vi "Vision Processing.vi"(4 "error in (no error)":errorcluster, 6 "CameraDevRef":T1) -> ()   [LabVIEW 2011]
uses:
  <vilib>/Rock Robotics/WPI/Camera/WPI_CameraDevRef.ctl
  Robot Global Data.vi
  <vilib>/vision/NI_Vision_Development_Module.lvlib
panel:
  in  "Y AbsolVal Difference":dbl=0.25
  in  "Default Shooter Speed Dump":dbl=0.42
  in  "Default Shooter Speed Shoot":dbl=0.705
  in  "Scale":dbl=0.85
  in  "Minimum Power":dbl=0.22
  out "Aspect Ratio":dbl[](array[numeric])
  out "Offset":dbl
  out "Raw Turret":dbl
  out "Target X Coord":dbl
  out "Target Distance":dbl
  out "Distance Array":dbl[](array[numeric])
  in  "Dead Band":dbl=0.09
  out "Number of Rectangles Visible":dbl
  out "Y Position Array":dbl[](array[numeric])
  out "X Position Array":dbl[](array[numeric])
  in  "View":bool
  out "Target Info":T2(array[cluster])
  in  "Area Size Limit":i32=444
  in  "Particle Count Limit":i32=8
  in  "Score Limits":T3={"Rect Coverage"=76.0, "Aspect Ratio"=40.0, "X Edge Strength"=40.0, "Y Edge Strength"=60.0}
  in  "Processing":enum32{"Color", "Intensity", "Intensity Open"}(tab)=enum."Intensity"
  in  "Luminance":i32=255
  in  "Saturation":i32=255
  in  "Hue":i32(knob)=65 scale=0.0..255.0
  in  "Margins":cluster{"Hue":i32, "Sat":i32, "Lum":i32}={"Hue"=20, "Sat"=27, "Lum"=30} {"Sat" scale=0.0..40.0; "Lum" scale=0.0..40.0; "Hue" scale=0.0..40.0}
  in  "Range":cluster{"Lower value":sgl, "Upper value":sgl}={"Lower value"=151.52174, "Upper value"=255.0} {"Lower value" scale=0.0..255.0; "Upper value" scale=0.0..255.0}
  in  "Range":cluster{"Lower value":sgl, "Upper value":sgl}={"Lower value"=123.804344, "Upper value"=255.0} {"Lower value" scale=0.0..255.0; "Upper value" scale=0.0..255.0}
  in  "View":bool
  out "Processed Image":T4(plugin-control)
  out "Original Image":T4(plugin-control)
  # "Instructions:\nProcessing the reflective tape that is illuminated by a ring light can be based\non color or light intensity.\nParticles within the image are scored by rectangle coverage, aspect ratio, and\nfor being hollow with a bold edge. A particle is considered a target if all scores\nare above the score limits. Particles can be annotated -- surrounded by\na rectangle and scores drawn to the left .\nTo control the number of particles being scored, use the count limit and the size\nlimit."
  # "(in)"
  # "To debug, Enable using the View button.\nFor color processing, you can click in the image to select the color for processing."
  # "Enable by clicking the View button.\nGreen scores are above the limit, orange are below. Inner/outer rect\nindicates all passed."
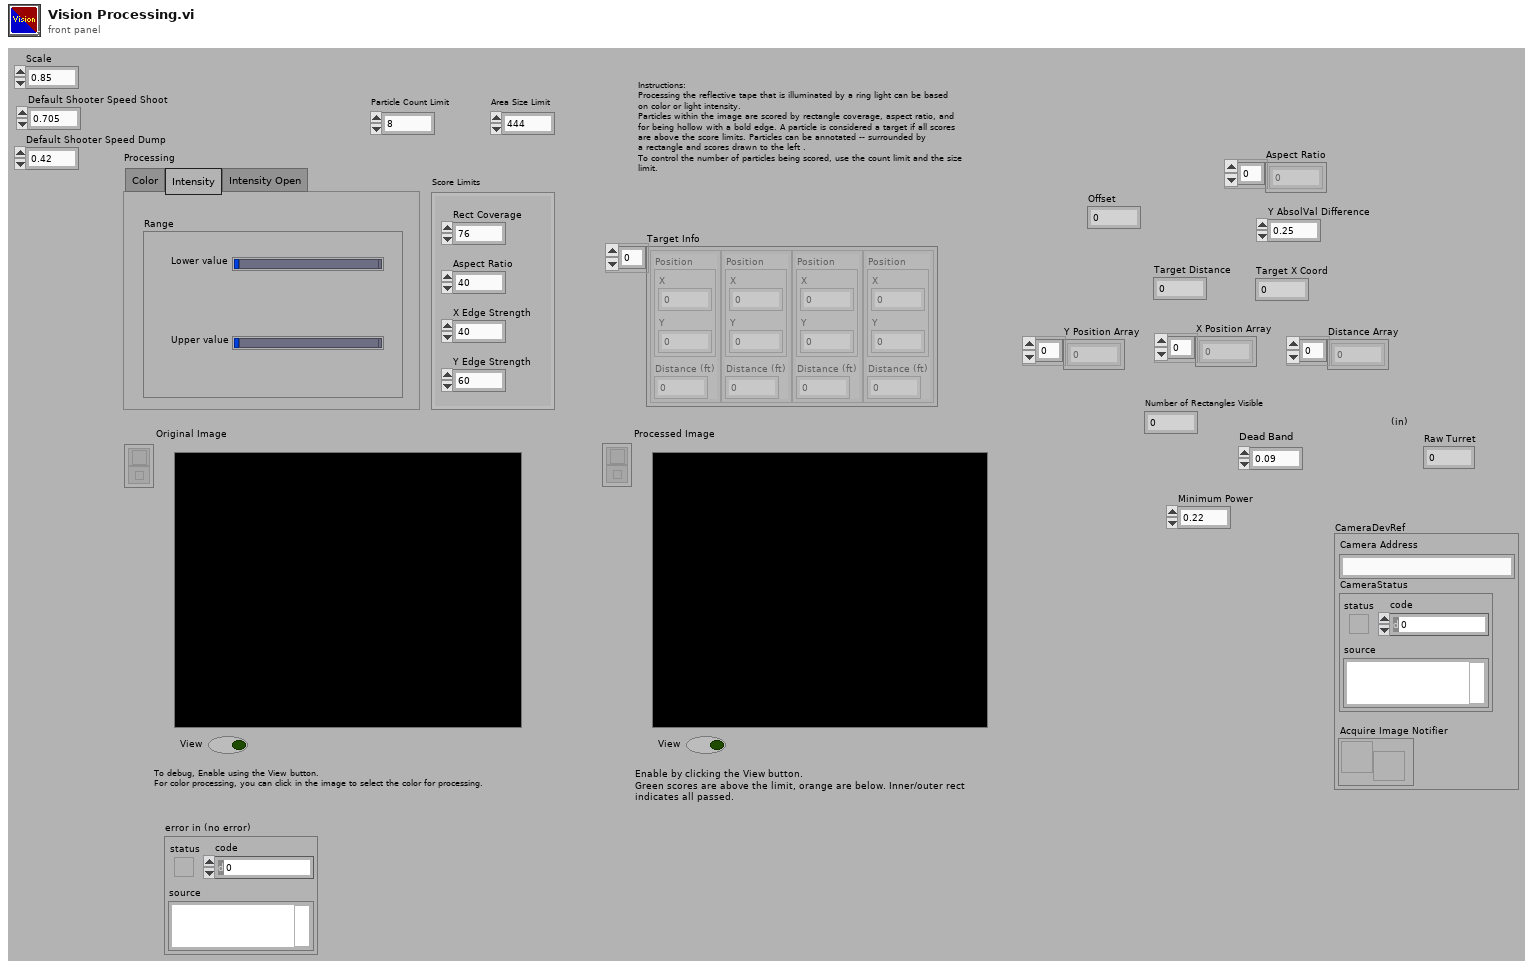
[diagram p1: front panel]
types:
  T1 = typedef "WPI_CameraDevRef.ctl" = cluster{"Camera Address":string, "CameraStatus":errorcluster, "Acquire Image Notifier":refnum<notifier>}
  T2 = cluster{"Position":cluster{"X":dbl, "Y":dbl}, "Distance (ft)":dbl}[]
  T3 = cluster{"Rect Coverage":dbl, "Aspect Ratio":dbl, "X Edge Strength":dbl, "Y Edge Strength":dbl}
  T4 = typedef "IMAQ Image.ctl" = refnum<image>
  T5 = typedef "Image Type" = u32
  T6 = enum32{"AutoM", "Close", "Dilate", "Erode", "Gradient", "Gradient out", "Gradient in", "Hit miss", "Open", "PClose", "POpen", "Thick", "Thin"}
  T7 = typedef "WPI_CameraImageSize.ctl" = enum16{"640x480", "320x240", "160x120"}
  T8 = cluster{"fps":i32, "compression":i32, "Image Size":T7}
  T9 = cluster{cluster{"Left":dbl, "Top":dbl, "Right":dbl, "Bottom":dbl}, dbl[]}[]
  T10 = cluster{"Left":dbl, "Top":dbl, "Right":dbl, "Bottom":dbl}
  T11 = cluster{"Target Center (-1 to 1)":cluster{"X":dbl, "Y":dbl}, "Distance (ft)":dbl}
  T12 = cluster{"Target Center (-1 to 1)":cluster{"X":dbl, "Y":dbl}, "Distance (ft)":dbl}[]
  T13 = typedef "WPI_JoystickDevRef.ctl" = cluster{"Device":T14}
  T14 = typedef "WPI_JoystickDeviceEnum.ctl" = enum16{"USB 1", "USB 2", "USB 3", "USB 4", "Kinect 1", "Kinect 2"}
  T15 = typedef "WPI_JoystickButtonState.ctl" = cluster{"Button 1":bool, "Button 2":bool, "Button 3":bool, "Button 4":bool, "Button 5":bool, "Button 6":bool, "Button 7":bool, "Button 8":bool, "Button 9":bool, "Button 10":bool, "Button 11":bool, "Button 12":bool}
  T16 = cluster{"axis 1 (x)":dbl, "axis 2 (y)":dbl, "axis 3 (throttle)":dbl, "axis 4":dbl, "axis 5":dbl, "axis 6":dbl}
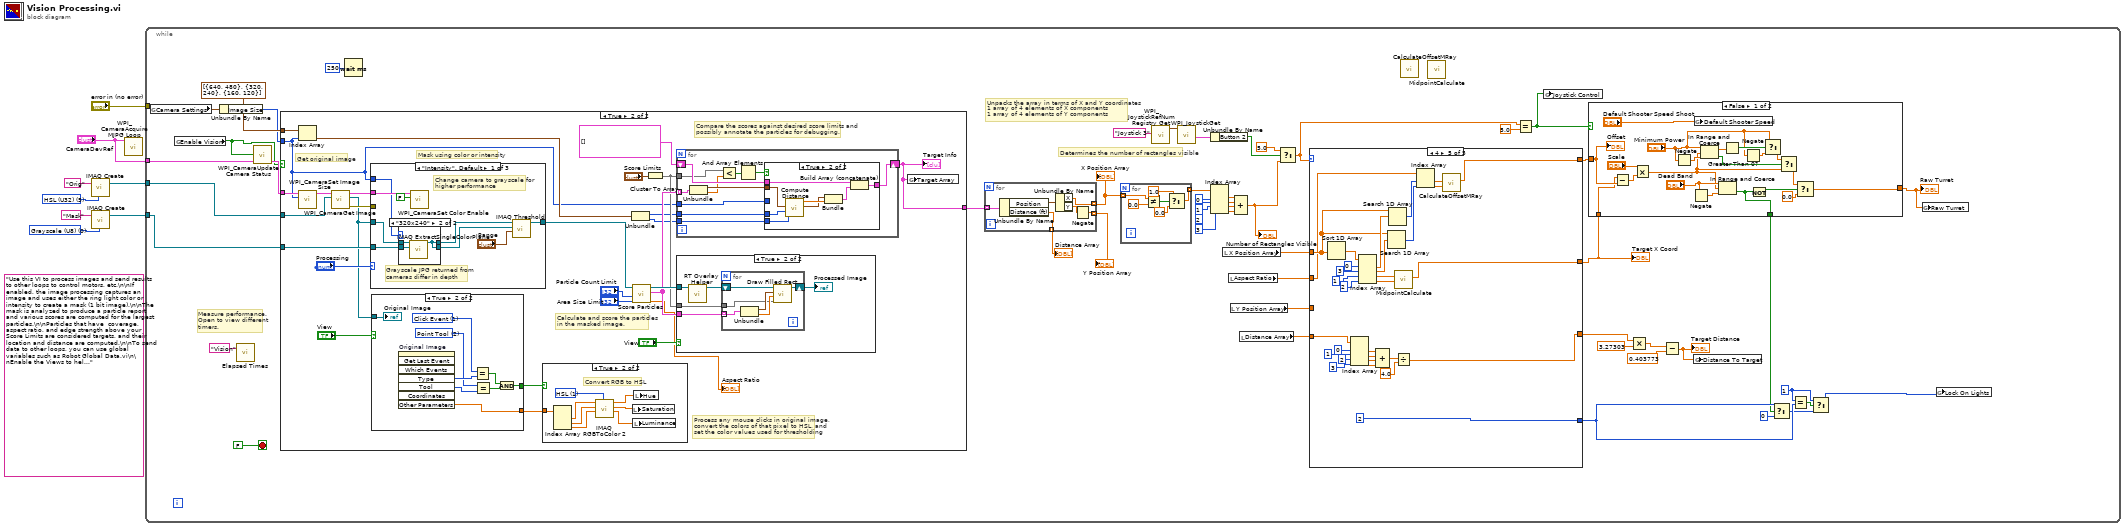
[diagram p0: block diagram]
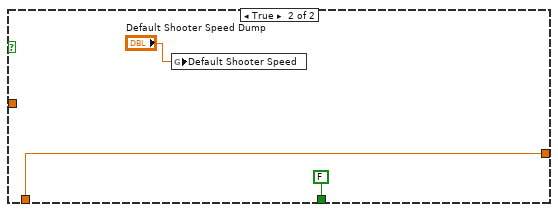
[diagram p2: hidden frame]
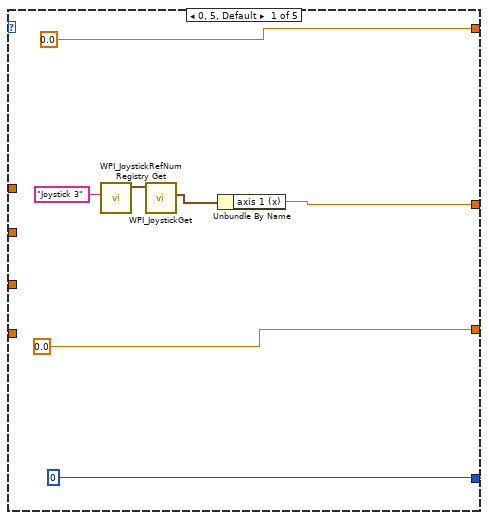
[diagram p3: hidden frame]
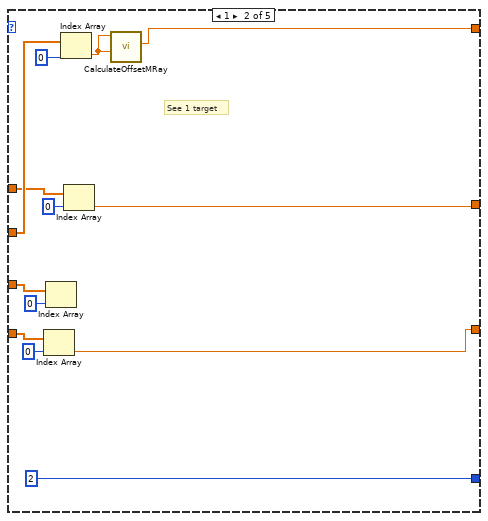
[diagram p4: hidden frame]
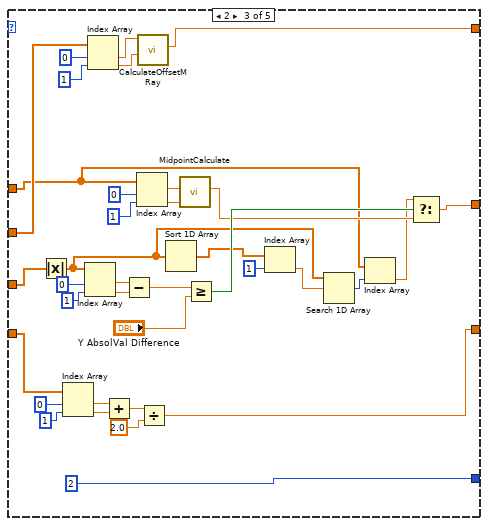
[diagram p5: hidden frame]
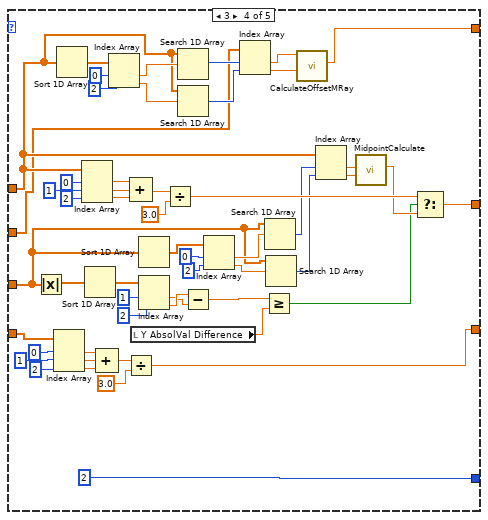
[diagram p6: hidden frame]
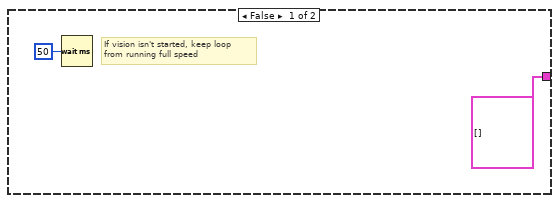
[diagram p7: hidden frame]
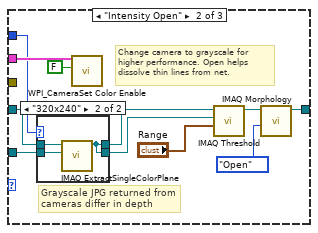
[diagram p10: hidden frame]
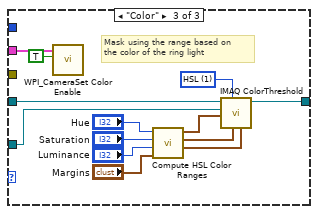
[diagram p12: hidden frame]
diagram:
  w3 = T5 0 items=["Grayscale (U8)", "Grayscale (I16)", "Grayscale (SGL)", "Complex (CSG)", "RGB (U32)", "HSL (U32)", "RGB (U64)", "Grayscale (U16)"] ("Image Type")
  (unwired) "Use this VI to process images and send results to other loops to control motors, etc.\n\nIf enabled, the image processing captures an image and uses either the ring light color or intensity to create a mask (1 bit image).\n\nThe mask is analyzed to produce a particle report and various scores are computed for the largest particles.\n\nParticles that have  coverage, aspect ratio, and edge strength above your Score Limits are considered targets, and their location and distance are computed.\n\nTo send data to other loops, you can use global variables such as Robot Global Data.vi\n\nEnable the Views to help debug color settings. Disable the View to speed up processing."
  w7 = T5 5 items=["Grayscale (U8)", "Grayscale (I16)", "Grayscale (SGL)", "Complex (CSG)", "RGB (U32)", "HSL (U32)", "RGB (U64)", "Grayscale (U16)"] ("Image Type")
  n1 = call "IMAQ Create"("Image Name"="Orig", "Image Type"=w7) -> ("New Image"=w6:T4)  [unwired: 2 in, 2 out]
  n2 = call "IMAQ Create"("Image Name"="Mask", "Image Type"=w3) -> ("New Image"=w1:T4)  [unwired: 2 in, 2 out]
  n3 = call <vilib>:"WPI_CameraAcquire MJPG Loop.vi"("CameraDevRef"="CameraDevRef") -> ()  [unwired: 11 in]
  n4 = while {
    tunnel: w6 -> [w59]
    tunnel: "CameraDevRef" -> [w58]
    tunnel: "error in (no error)" -> [_]
    tunnel: w1 -> [w54]
    stop <- FALSE stop-if-true
    w24 = 1 ("y")
    # "Determines the number of rectangles visible"
    # "Unpacks the array in terms of X and Y coordinates\n1 array of 4 elements of X components\n1 array of 4 elements of Y components"
    # "Measure performance.\nOpen to view different\ntimers."
    n5 = global read "Robot Global Data.vi" "Camera Settings"() -> (w52:T8)
    n6 = global read "Robot Global Data.vi" "Enable Vision"() -> (w56:bool)
    n7 = Unbundle By Name(w52) -> ("Image Size"=w51:T7)
    n8 = call "Elapsed Times.vi"("Call Name"="Vision") -> ()  [unwired: 2 in, 1 out]
    n9 = call <vilib>:"WPI_CameraUpdate Camera Status.vi"("CameraDevRef In"=w58, "Enable Vision"=w56) -> ("CameraDevRef Out"=w57:T1)  [unwired: 3 in]
    n10 = case shown="True" w56 {
      tunnel: w59 -> [_ w254]
      tunnel: w57 -> [_ w250]
      tunnel: w54 -> [_ w241]
      tunnel: cluster{i32, i32}[] [{640, 480}, {320, 240}, {160, 120}] -> [_ w245]
      tunnel: w51 -> [_ w238]
      tunnel: [T2 [] w239] -> w50
      frame False {
        # "If vision isn't started, keep loop\nfrom running full speed"
        n11 = Wait (ms)(milliseconds to wait=u32 50) -> ()  [unwired: 1 out]
      }
      frame True {
        # "Compare the scores against desired score limits and\npossibly annotate the particles for debugging."
        # "Process any mouse clicks in original image,\nconvert the colors of that pixel to HSL, and\nset the color values used for thresholding"
        # "Calculate and score the particles\nin the masked image."
        # "Mask using color or intensity"
        # "Get original image"
        n12 = call <vilib>:"WPI_CameraSet Image Size.vi"("Image Size"=w238, "CameraDevRef"=w250) -> ("CameraDevRef Out"=w251:T1)  [unwired: 8 in, 1 out]
        n13 = Index Array(array=w245, index=w238) -> (element=w242:cluster{i32, i32})
        n14 = call <vilib>:"WPI_CameraGet Image.vi"("Image"=w254, "CameraDevRef"=w251) -> ("error out"=w252:errorcluster, "Image Out"=w240:T4, "CameraDevRef Out"=w253:T1)  [unwired: 7 in]
        n15 = case shown="\"Intensity\", Default" "Processing" {
          tunnel: w240 -> [w276 w288 w314]
          tunnel: [w279 w293 w313] -> w248
          tunnel: w253 -> [w277 w291 w304]
          tunnel: w252 -> [_ _ _]
          tunnel: w241 -> [w275 w289 w302]
          tunnel: w238 -> [w274 w290 _]
          frame "Intensity", Default {
            # "Grayscale JPG returned from\ncameras differ in depth"
            # "Change camera to grayscale for\nhigher performance"
            n16 = case shown="\"320x240\"" w274 {
              tunnel: w276 -> [w282 w285]
              tunnel: w275 -> [w281 w284]
              tunnel: [w282 w283] -> w273
              tunnel: [w281 w283] -> w272
              frame "640x480", Default {
              }
              frame "320x240" {
                n17 = call "IMAQ ExtractSingleColorPlane"("Image Dst"=w284, "Image Src"=w285) -> ("Image Dst Out"=w283:T4)  [unwired: 8 in, 1 out]
              }
            }
            n18 = call <vilib>:"WPI_CameraSet Color Enable.vi"("Color Enabled"=FALSE, "CameraDevRef"=w277) -> ()  [unwired: 8 in, 2 out]
            n19 = call "IMAQ Threshold"("Range"="Range", "Image Dst"=w272, "Image Src"=w273) -> ("Image Dst Out"=w279:T4)  [unwired: 3 in, 5 out]
          }
          frame "Intensity Open" {
            # "Grayscale JPG returned from\ncameras differ in depth"
            # "Change camera to grayscale for\nhigher performance. Open helps\ndissolve thin lines from net."
            n20 = case shown="\"320x240\"" w290 {
              tunnel: w288 -> [w298 w301]
              tunnel: w289 -> [w297 w300]
              tunnel: [w298 w299] -> w287
              tunnel: [w297 w299] -> w286
              frame "640x480", Default {
              }
              frame "320x240" {
                n21 = call "IMAQ ExtractSingleColorPlane"("Image Dst"=w300, "Image Src"=w301) -> ("Image Dst Out"=w299:T4)  [unwired: 8 in, 1 out]
              }
            }
            n22 = call <vilib>:"WPI_CameraSet Color Enable.vi"("Color Enabled"=FALSE, "CameraDevRef"=w291) -> ()  [unwired: 8 in, 2 out]
            n23 = call "IMAQ Threshold"("Range"="Range", "Image Dst"=w286, "Image Src"=w287) -> ("Image Dst Out"=w294:T4)  [unwired: 3 in, 5 out]
            n24 = call "IMAQ Morphology"("Operation"=T6."Open", "Image Src"=w294) -> ("Image Dst Out"=w293:T4)  [unwired: 8 in, 1 out]
          }
          frame "Color" {
            w312 = u16 1 items=["RGB", "HSL", "HSV", "HSI"] ("Color Mode")
            # "Mask using the range based on\nthe color of the ring light"
            n25 = call <vilib>:"WPI_CameraSet Color Enable.vi"("Color Enabled"=TRUE, "CameraDevRef"=w304) -> ()  [unwired: 8 in, 2 out]
            n26 = call "Compute HSL Color Ranges.vi"("Margins"="Margins", "Luminance"="Luminance", "Saturation"="Saturation", "Hue"="Hue") -> ("Lum Range"=w309:cluster{i32, i32}, "Sat Range"=w310:cluster{i32, i32}, "Hue Range"=w311:cluster{i32, i32})  [unwired: 5 in]
            n27 = call "IMAQ ColorThreshold"("Blue or Luma or Val or Inten Range"=w309, "Green or Sat Range"=w310, "Color Mode"=w312, "Red or Hue Range"=w311, "Image Dst"=w302, "Image Src"=w314) -> ("Image Dst Out"=w313:T4)  [unwired: 4 in, 1 out]
          }
        }
        n28 = case shown="True" "View" {
          tunnel: w240 -> [_ w334]
          tunnel: [_ w329] -> w247
          tunnel: [_ w326] -> w246
          frame False {
          }
          frame True {
            w327 = 2 items=["None", "Selection Tool", "Point Tool", "Line Tool", "Rectangle Tool", "Oval Tool", "Polygon Tool", "ClosedFreehandTool", "Annulus Tool", "Rotated Rectangle Tool", "Zoom Tool", "Pan Tool", "Polyline Tool", "Freehand Tool"] ("Tool")
            w328 = 1 items=["No Event"=0, "Click Event"=1, "Draw Event"=2, "Size Event"=4, "Scroll Event"=5, "Double Click Event"=8] ("Type")
            n29 = invoke on="Original Image" class="ImageControl" method="Get Last Event"() -> ("Type"=w330:i32, "Tool"=w333:i32, "Other Parameters"=w326:sgl[])  [unwired: 8 in, 5 out]
            n30 = Equal?(x=w328, y=w330) -> (x = y?=w331:bool)
            n31 = Equal?(x=w327, y=w333) -> (x = y?=w332:bool)
            n32 = And(x=w331, y=w332) -> (x .and. y?=w329:bool)
            "Original Image" <- w334
          }
        }
        n33 = case shown="True" w247 {
          tunnel: w246 -> [_ w271]
          frame False {
          }
          frame True {
            w270 = u16 1 items=["RGB", "HSL", "HSV", "HSI", "CIE L*a*b*", "CIE XYZ"] ("Color Mode")
            # "Convert RGB to HSL"
            n34 = Index Array(array=w271) -> (element #1=w269:sgl, element #2=w267:sgl, element #3=w265:sgl)  [unwired: 3 in]
            n35 = call "IMAQ RGBToColor 2"("Color Mode"=w270, "Blue value"=w265, "Green value"=w267, "Red value"=w269) -> ("Blue or Luma or Val or Inten or Z or b*value"=w264:dbl, "Green or Sat or Y or a* value"=w266:dbl, "Red or Hue or X or L* value"=w268:dbl)  [unwired: 4 in, 1 out]
            n36 = local write "Saturation"(w266) -> ()
            n37 = local write "Luminance"(w264) -> ()
            n38 = local write "Hue"(w268) -> ()
          }
        }
        n39 = Unbundle(w242) -> (w244:i32, w243:i32)
        n40 = call "Score Particles.vi"("Area Size Limit"="Area Size Limit", "Particle Count Limit"="Particle Count Limit", "Image Refnum in"=w248) -> ("Aspect Ratio"=→"Aspect Ratio":dbl[], "Scored Particle Info"=w259:T9, "Image Refnum out"=w262:T4)  [unwired: 6 in]
        n41 = Cluster To Array(cluster="Score Limits") -> (array=w257:dbl[])
        n42 = for {
          shift-right: [w344] -> w239
          shift-left: T2 [] -> [w345]
          tunnel: w244 -> [w343]
          tunnel: w259 -> [w341] mode=indexing
          tunnel: w257 -> [w336]
          tunnel: w238 -> [w340]
          tunnel: w243 -> [w335]
          n43 = Unbundle(w341) -> (w342:T10, w337:dbl[])
          n44 = Less?(x=w336, y=w337) -> (x < y?=w339:bool[])
          n45 = And Array Elements(Boolean array=w339) -> (logical AND=w338:bool)
          n46 = case shown="True" w338 {
            tunnel: w345 -> [w346 w354]
            tunnel: [w346 w353] -> w344
            tunnel: w342 -> [_ w349]
            tunnel: w343 -> [_ w351]
            tunnel: w340 -> [_ _]
            tunnel: w335 -> [_ w348]
            frame False {
            }
            frame True {
              n47 = call "Compute Distance.vi"("Y Image Resolution"=w348, "X Image Resolution"=w351, "Bounding Box"=w349) -> ("Target Center (-1 to 1)"=w347:cluster{"X":dbl, "Y":dbl}, "Distance (ft)"=w350:dbl)  [unwired: 7 in]
              n48 = Bundle("Target Center (-1 to 1)"=w347, "Distance (ft)"=w350) -> (w352:T11)  [unwired: 1 in]
              n49 = Build Array (concatenate)(w354, w352) -> (w353:T12)
            }
          }
        }
        "Target Info" <- w239
        n50 = case shown="True" "View" {
          tunnel: w262 -> [_ w316]
          tunnel: w259 -> [_ w318]
          tunnel: w257 -> [_ w317]
          frame False {
          }
          frame True {
            n51 = call "RT Overlay Helper.vi"("Refnum in"=w316) -> ("Refnum out"=w319:T4)  [unwired: 10 in]
            n52 = for {
              shift-right: [w324] -> w315
              shift-left: w319 -> [w325]
              tunnel: w318 -> [w321] mode=indexing
              tunnel: w317 -> [w320]
              n53 = Unbundle(w321) -> (w322:T10, w323:dbl[])
              n54 = call "Draw Filled Rect.vi"("Limits"=w320, "Scores"=w323, "Bounding Box"=w322, "image in"=w325) -> ("image out"=w324:T4)  [unwired: 7 in]
            }
            "Processed Image" <- w315
          }
        }
        n55 = global write "Robot Global Data.vi" "Target Array"(w239) -> ()
      }
    }
    n56 = Wait (ms)(milliseconds to wait=u32 250) -> ()  [unwired: 1 out]
    n57 = for {
      tunnel: [w232] -> w30 mode=indexing
      tunnel: [w233] -> w40 mode=indexing
      tunnel: w50 -> [w230] mode=indexing
      tunnel: [w229] -> w42 mode=indexing
      n58 = Unbundle By Name(w230) -> ("Position"=w234:cluster{"X":dbl, "Y":dbl}, "Distance (ft)"=w229:dbl)
      n59 = Unbundle By Name(w234) -> ("X"=w233:dbl, "Y"=w231:dbl)
      n60 = Negate(x=w231) -> (-x=w232:dbl)
    }
    "X Position Array" <- w40
    "Y Position Array" <- w30
    "Distance Array" <- w42
    n61 = for {
      tunnel: w40 -> [w88] mode=indexing
      tunnel: [w84] -> w39 mode=indexing
      n62 = Not Equal?(x=w88, y=0.0) -> (x != y?=w87:bool)
      n63 = Select(t=1.0, s=w87, f=0.0) -> (s? t:f=w84:dbl)
    }
    n64 = call <vilib>:"WPI_JoystickRefNum Registry Get.vi"("refnum name"="Joystick 3") -> ("JoystickDevRef"=w29:T13)  [unwired: 9 in, 1 out]
    n65 = call <vilib>:"WPI_JoystickGet.vi"("JoystickDevRef"=w29) -> ("Buttons"=w27:T15)  [unwired: 4 in, 2 out]
    n66 = Unbundle By Name(w27) -> ("Button 2"=w26:bool)
    n67 = Index Array(array=w39, index #1=0 ("index"), index #2=1 ("index"), index #3=2 ("index"), index #4=3 ("index")) -> (element #1=w37:dbl, element #2=w38:dbl, element #3=w36:dbl, element #4=w35:dbl)
    n68 = local read "X Position Array"() -> (w41:dbl[])
    n69 = local read "Aspect Ratio"() -> (w19:dbl[])
    n70 = local read "Y Position Array"() -> (w43:dbl[])
    n71 = Compound Arithmetic op=ADD(w37, w38, w36, w35) -> (w20:dbl)
    "Number of Rectangles Visible" <- w20
    n72 = local read "Distance Array"() -> (w44:dbl[])
    n73 = Select(t=5.0, s=w26, f=w20) -> (s? t:f=w14:dbl)
    n74 = case shown="4" w14 {
      tunnel: w41 -> [_ w104 w111 w153 w204]
      tunnel: [w92 w103 w135 w187 w227] -> w17
      tunnel: w43 -> [_ w101 w134 w165 _]
      tunnel: w44 -> [_ w99 w123 w196 w224]
      tunnel: [0 2 2 2 2] -> w23
      tunnel: [0.0 ("Offset") w106 w140 w146 w213] -> w18
      tunnel: w19 -> [_ w109 w143 w149 w199]
      tunnel: [0.0 w98 w118 w189 w214] -> w9
      frame 0, 5, Default {
        n75 = call <vilib>:"WPI_JoystickRefNum Registry Get.vi"("refnum name"="Joystick 3") -> ("JoystickDevRef"=w91:T13)  [unwired: 9 in, 1 out]
        n76 = call <vilib>:"WPI_JoystickGet.vi"("JoystickDevRef"=w91) -> ("Axes"=w93:T16)  [unwired: 4 in, 2 out]
        n77 = Unbundle By Name(w93) -> ("axis 1 (x)"=w92:dbl)
      }
      frame 1 {
        # "See 1 target"
        n78 = Index Array(array=w99, index=0) -> (element=w98:dbl)
        n79 = Index Array(array=w101, index=0) -> ()  [unwired: 1 out]
        n80 = Index Array(array=w109, index=0) -> (element=w107:dbl)
        n81 = Index Array(array=w104, index=0) -> (element=w103:dbl)
        n82 = call "CalculateOffsetMRay.vi"("AR2"=w107, "AR1"=w107) -> ("Offset"=w106:dbl)  [unwired: 9 in]
      }
      frame 2 {
        n83 = Absolute Value(x=w134) -> (abs(x)=w114:dbl[])
        n84 = Index Array(array=w123, index #1=0 ("index"), index #2=1 ("index")) -> (element #1=w121:dbl, element #2=w122:dbl)
        n85 = Index Array(array=w114, index #1=0 ("index"), index #2=1 ("index")) -> (element #1=w130:dbl, element #2=w131:dbl)
        n86 = Index Array(array=w143, index #1=0 ("index"), index #2=1 ("index")) -> (element #1=w142:dbl, element #2=w141:dbl)
        n87 = Add(x=w121, y=w122) -> (x+y=w120:dbl)
        n88 = Subtract(x=w130, y=w131) -> (x-y=w129:dbl)
        n89 = Index Array(array=w111, index #1=0 ("index"), index #2=1 ("index")) -> (element #1=w136:dbl, element #2=w137:dbl)
        n90 = call "CalculateOffsetMRay.vi"("AR2"=w141, "AR1"=w142) -> ("Offset"=w140:dbl)  [unwired: 9 in]
        n91 = Divide(x=w120, y=2.0) -> (x/y=w118:dbl)
        n92 = Sort 1D Array(array=w114) -> (sorted array=w116:dbl[])
        n93 = call "MidpointCalculate.vi"("X2"=w137, "X1"=w136) -> ("Midpoint"=w126:dbl)  [unwired: 9 in]
        n94 = Greater Or Equal?(x=w129, y="Y AbsolVal Difference") -> (x >= y?=w127:bool)
        n95 = Index Array(array=w116, index=1) -> (element=w113:dbl)
        n96 = Search 1D Array(1D array=w114, element=w113) -> (index of element=w112:i32)  [unwired: 1 in]
        n97 = Index Array(array=w111, index=w112) -> (element=w110:dbl)
        n98 = Select(t=w110, s=w127, f=w126) -> (s? t:f=w135:dbl)
      }
      frame 3 {
        n99 = Absolute Value(x=w165) -> (abs(x)=w186:dbl[])
        n100 = Index Array(array=w196, index #1=0 ("index"), index #2=1 ("index"), index #3=2 ("index")) -> (element #1=w192:dbl, element #2=w193:dbl, element #3=w194:dbl)
        n101 = Sort 1D Array(array=w153) -> (sorted array=w157:dbl[])
        n102 = Index Array(array=w153, index #1=0 ("index"), index #2=1 ("index"), index #3=2 ("index")) -> (element #1=w174:dbl, element #2=w176:dbl, element #3=w175:dbl)
        n103 = Sort 1D Array(array=w186) -> (sorted array=w170:dbl[])
        n104 = Compound Arithmetic op=ADD(w192, w193, w194) -> (w191:dbl)
        n105 = Index Array(array=w157, index #1=0 ("index"), index #2=2 ("index")) -> (element #1=w154:dbl, element #2=w152:dbl)
        n106 = Divide(x=w191, y=3.0) -> (x/y=w189:dbl)
        n107 = Compound Arithmetic op=ADD(w174, w176, w175) -> (w173:dbl)
        n108 = local read "Y AbsolVal Difference"() -> (w180:dbl)
        n109 = Sort 1D Array(array=w165) -> (sorted array=w169:dbl[])
        n110 = Index Array(array=w170, index #1=1 ("index"), index #2=2 ("index")) -> (element #1=w182:dbl, element #2=w183:dbl)
        n111 = Divide(x=w173, y=3.0) -> (x/y=w171:dbl)
        n112 = Search 1D Array(1D array=w153, element=w154) -> (index of element=w151:i32)  [unwired: 1 in]
        n113 = Search 1D Array(1D array=w153, element=w152) -> (index of element=w150:i32)  [unwired: 1 in]
        n114 = Subtract(x=w183, y=w182) -> (x-y=w181:dbl)
        n115 = Index Array(array=w169, index #1=0 ("index"), index #2=2 ("index")) -> (element #1=w166:dbl, element #2=w164:dbl)
        n116 = Index Array(array=w149, index #1=w151, index #2=w150) -> (element #1=w148:dbl, element #2=w147:dbl)
        n117 = Greater Or Equal?(x=w181, y=w180) -> (x >= y?=w158:bool)
        n118 = Search 1D Array(1D array=w165, element=w166) -> (index of element=w163:i32)  [unwired: 1 in]
        n119 = Search 1D Array(1D array=w165, element=w164) -> (index of element=w162:i32)  [unwired: 1 in]
        n120 = call "CalculateOffsetMRay.vi"("AR2"=w147, "AR1"=w148) -> ("Offset"=w146:dbl)  [unwired: 9 in]
        n121 = Index Array(array=w153, index #1=w163, index #2=w162) -> (element #1=w160:dbl, element #2=w161:dbl)
        n122 = call "MidpointCalculate.vi"("X2"=w161, "X1"=w160) -> ("Midpoint"=w159:dbl)  [unwired: 9 in]
        n123 = Select(t=w171, s=w158, f=w159) -> (s? t:f=w187:dbl)
      }
      frame 4 {
        n124 = Sort 1D Array(array=w204) -> (sorted array=w228:dbl[])
        n125 = Index Array(array=w224, index #1=0 ("index"), index #2=1 ("index"), index #3=2 ("index"), index #4=3 ("index")) -> (element #1=w221:dbl, element #2=w220:dbl, element #3=w219:dbl, element #4=w218:dbl)
        n126 = Index Array(array=w228, index #1=0 ("index"), index #2=3 ("index"), index #3=1 ("index"), index #4=2 ("index")) -> (element #1=w205:dbl, element #2=w206:dbl, element #3=w212:dbl, element #4=w211:dbl)
        n127 = Compound Arithmetic op=ADD(w221, w220, w219, w218) -> (w217:dbl)
        n128 = Search 1D Array(1D array=w204, element=w206) -> (index of element=w201:i32)  [unwired: 1 in]
        n129 = Search 1D Array(1D array=w204, element=w205) -> (index of element=w200:i32)  [unwired: 1 in]
        n130 = call "MidpointCalculate.vi"("X2"=w211, "X1"=w212) -> ("Midpoint"=w227:dbl)  [unwired: 9 in]
        n131 = Divide(x=w217, y=4.0) -> (x/y=w214:dbl)
        n132 = Index Array(array=w199, index #1=w200, index #2=w201) -> (element #1=w203:dbl, element #2=w202:dbl)
        n133 = call "CalculateOffsetMRay.vi"("AR2"=w202, "AR1"=w203) -> ("Offset"=w213:dbl)  [unwired: 9 in]
      }
    }
    "Target X Coord" <- w17
    n134 = call "CalculateOffsetMRay.vi"() -> ()  [unwired: 11 in, 1 out]
    n135 = call "MidpointCalculate.vi"() -> ()  [unwired: 11 in, 1 out]
    n136 = Equal?(x=w14, y=5.0) -> (x = y?=w10:bool)
    n137 = global write "Robot Global Data.vi" "Joystick Control"(w10) -> ()
    n138 = case shown="False" w10 {
      tunnel: w18 -> [w79 _]
      tunnel: w17 -> [w78 w83]
      tunnel: [w61 w83] -> w48
      tunnel: [w64 FALSE] -> w16
      frame False {
        n139 = Subtract(x=w78, y=w79) -> (x-y=w76:dbl)
        n140 = Multiply(x="Scale", y=w76) -> (x*y=w67:dbl)
        n141 = Negate(x="Minimum Power") -> (-x=w74:dbl)
        n142 = Negate(x="Dead Band") -> (-x=w80:dbl)
        n143 = global write "Robot Global Data.vi" "Default Shooter Speed"("Default Shooter Speed Shoot") -> ()
        n144 = In Range and Coerce(upper limit="Minimum Power", x=w67, lower limit=w74) -> (coerced(x)=w70:dbl, In Range?=w71:bool)
        n145 = In Range and Coerce(upper limit="Dead Band", x=w67, lower limit=w80) -> (In Range?=w64:bool)  [unwired: 1 out]
        n146 = Greater Than 0?(x=w70) -> (x > 0?=w69:bool)
        n147 = Negate(x="Minimum Power") -> (-x=w66:dbl)
        n148 = Not(x=w64) -> (.not. x?=w65:bool)
        n149 = Select(t="Minimum Power", s=w69, f=w66) -> (s? t:f=w68:dbl)
        n150 = Select(t=w68, s=w71, f=w67) -> (s? t:f=w72:dbl)
        n151 = Select(t=w72, s=w65, f=0.0) -> (s? t:f=w61:dbl)
        "Offset" <- w79
      }
      frame True {
        n152 = global write "Robot Global Data.vi" "Default Shooter Speed"("Default Shooter Speed Dump") -> ()
      }
    }
    "Raw Turret" <- w48
    n153 = Multiply(x=w9, y=3.27303) -> (x*y=w13:dbl)
    n154 = Subtract(x=w13, y=0.403773) -> (x-y=w46:dbl)
    "Target Distance" <- w46
    n155 = global write "Robot Global Data.vi" "Distance To Target"(w46) -> ()
    n156 = Select(t=w23, s=w16, f=0) -> (s? t:f=w21:i32)
    n157 = Equal?(x=w24, y=w23) -> (x = y?=w25:bool)
    n158 = Select(t=w24, s=w25, f=w21) -> (s? t:f=w47:i32)
    n159 = global write "Robot Global Data.vi" "Raw Turret"(w48) -> ()
    n160 = global write "Robot Global Data.vi" "Lock On Lights"(w47) -> ()
  }
